vi "writeData.vi"(0 "Buffer Num":u8, 1 "Buffer Addr":u8 format="%x", 2 "Frames to Write":u8, 3 "Data to Write":u8[](array[numeric])=[0, 0, 0, 0, 0, 0, 0, 0], 4 "SPI Config In":T1) -> (5 "SPI Config Out":T1)   [LabVIEW 2019]
uses:
  SPI/SPI Config.ctl
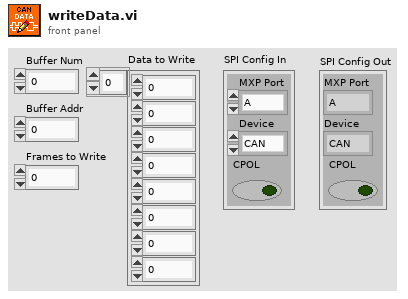
[diagram p1: front panel]
types:
  T1 = typedef "SPI Config.ctl" = cluster{"MXP Port":enum16{"A", "B"}, "Device":enum16{"CAN", "ENC", "IMU1", "IMU2"}, "CPOL":bool}
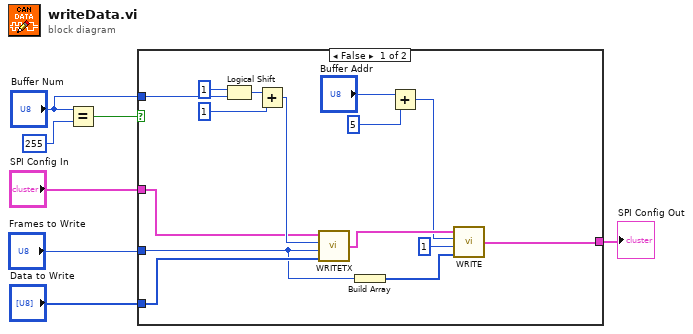
[diagram p0: block diagram]
diagram:
  n1 = Equal?(x="Buffer Num", y=u8 255) -> (x = y?=w6:bool)
  n2 = case shown="False" w6 {
    tunnel: "Buffer Num" -> [w8 _]
    tunnel: "Data to Write" -> [w17 _]
    tunnel: "SPI Config In" -> [w15 w23]
    tunnel: "Frames to Write" -> [w14 _]
    tunnel: [w10 w23] -> w1
    frame False {
      n3 = Logical Shift(y=i16 1, x=w8) -> (x << y=w21:u8)
      n4 = Add(x=w21, y=u8 1) -> (x+y=w16:u8)
      n5 = call "WRITETX.vi"("Data to Write"=w17, "Frames to Write"=w14, "Reg. Select"=w16, "SPI Config In"=w15) -> ("SPI Config Out"=w13:T1)
      n6 = Build Array(w14) -> (w12:u8[])
      n7 = Add(x="Buffer Addr", y=u8 5) -> (x+y=w11:u8)
      n8 = call "WRITE.vi"("Data to Write"=w12, "Frames to Write"=u8 1, "Starting Address"=w11, "SPI Config In"=w13) -> ("SPI Config Out"=w10:T1)
    }
    frame True {
    }
  }
  "SPI Config Out" <- w1
